vi "Data_SetEventRef.vi"(8 "error in (no error)":errorcluster, 10 "SendEventRef":T1) -> (0 "error out":errorcluster, 1 "ExtraLargeFile":bool, 2 "stream":bool, 3 "data":variant)   [LabVIEW 2017, in "FileManager.lvlib"]
uses:
  <vilib>/addons/InsightCM/Devices/Shared/Common/FileManager/FileManager.lvlib
  <vilib>/addons/InsightCM/Devices/Shared/Common/FileManager/controls/SendEventRefRoutedMessage.ctl
  <vilib>/addons/InsightCM/Devices/Shared/Common/DataEvent/controls/EventReference.ctl
  <vilib>/addons/InsightCM/Devices/Shared/Common/DataEvent/controls/Event.ctl
  <vilib>/addons/InsightCM/MessageBus/Base/controls/DataEvent.ctl
  <vilib>/addons/InsightCM/MessageBus/Base/controls/KeyValuePair.ctl
  <vilib>/addons/InsightCM/Devices/Shared/Common/DataEvent/controls/DataSet.ctl
  <vilib>/addons/InsightCM/MessageBus/Base/controls/DataSetMetadata.ctl
  <vilib>/addons/InsightCM/MessageBus/Base/controls/TrendPoint.ctl
  <vilib>/addons/InsightCM/MessageBus/Base/controls/TrendAlarmUpdate.ctl
  <vilib>/addons/InsightCM/MessageBus/Base/controls/TrendAlarmTransition.ctl
  <vilib>/addons/InsightCM/Devices/Shared/Common/FileManager/controls/DataPropertyNames.ctl
  <vilib>/addons/InsightCM/Devices/Shared/Common/FileManager/controls/DataType.ctl
  <vilib>/addons/InsightCM/Devices/Shared/Common/DataEvent/DataEvent.lvlib
panel:
  out "trend points only":bool
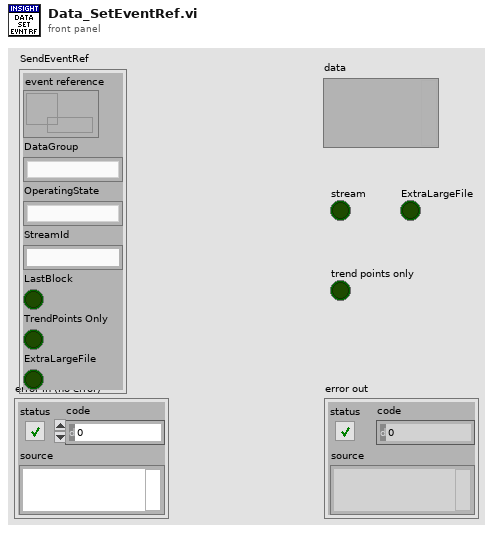
[diagram p1: front panel]
types:
  T1 = typedef "FileManager.lvlib/SendEventRefRoutedMessage.ctl" = cluster{"event reference":T2, "DataGroup":string, "OperatingState":string, "StreamId":string, "LastBlock":bool, "TrendPoints Only":bool, "ExtraLargeFile":bool}
  T2 = typedef "DataEvent.lvlib/EventReference.ctl" = refnum<data-value>
  T3 = typedef "DataPropertyNames.ctl" = enum16{"Type", "EventRef", "FilePath", "DataGroup", "AcquisitionTimestamp", "StreamId", "StreamBlock", "TrendPointsOnly", "ExtraLargeFile"}
  T4 = typedef "FileManager.lvlib/DataType.ctl" = enum16{"Default", "File", "InMemory", "EventRef", "EventRefFile"}
  T5 = typedef "DataEvent.lvlib/Event.ctl" = cluster{"DataEvent":T6, "DataSets":T8[], "TrendPoints":T10[], "Alarms":T11[]}
  T6 = typedef "DataEvent.ctl" = cluster{"Id":string, "AssetNodeId":string, "Timestamp":i64, "Props":T7[]}
  T7 = typedef "KeyValuePair.ctl" = cluster{"Key":string, "Value":string}
  T8 = typedef "DataEvent.lvlib/DataSet.ctl" = cluster{"DataSetMetadata":T9, "Values":sgl[], "Values DVR":refnum<data-value>}
  T9 = typedef "DataSetMetadata.ctl" = cluster{"Id":string, "DataEventId":string, "AssetNodeId":string, "Type":string, "T0":i64, "Props":T7[]}
  T10 = typedef "TrendPoint.ctl" = cluster{"TrendPointId":string, "DataEventId":string, "Timestamp":i64, "Value":dbl, "Props":T7[]}
  T11 = typedef "TrendAlarmUpdate.ctl" = cluster{"RuleId":string, "Transition":T12}
  T12 = typedef "TrendAlarmTransition.ctl" = cluster{"At":i64, "Severity":i32, "Value":dbl, "Properties":T7[]}
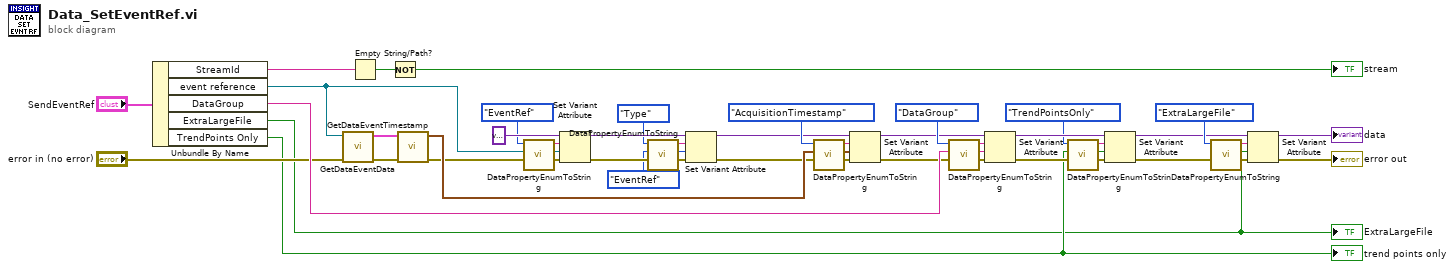
[diagram p0: block diagram]
diagram:
  n1 = Unbundle By Name("SendEventRef") -> ("StreamId"=w27:string, "event reference"=w21:T2, "DataGroup"=w33:string, "ExtraLargeFile"=w1:bool, "TrendPoints Only"=w2:bool)
  "trend points only" <- w2
  "ExtraLargeFile" <- w1
  n2 = call <vilib>:"GetDataEventData.vi"("error in (no error)"="error in (no error)", "Data Value Reference in"=w21) -> ("error out"=w22:errorcluster, "Data"=w20:T5)  [unwired: 8 in]
  n3 = Empty String/Path?(string/path=w27) -> (empty?=w26:bool)
  n4 = Not(x=w26) -> (.not. x?=→"stream":bool)
  n5 = call <vilib>:"GetDataEventTimestamp.vi"("error in (no error)"=w22, "data event"=w20) -> ("error out"=w24:errorcluster, "acquisition timestamp"=w30:timestamp)  [unwired: 8 in]
  n6 = call <vilib>:"DataPropertyEnumToString.vi"("property"=DataPropertyNames."EventRef" ("Names")) -> ("string"=w36:string)  [unwired: 10 in]
  n7 = Set Variant Attribute(Variant=variant ("DataInProgress"), name=w36, value=w21, error in=w24) -> (Variant out=w16:variant, error out=w19:errorcluster)  [unwired: 1 out]
  n8 = call <vilib>:"DataPropertyEnumToString.vi"("property"=DataPropertyNames."Type") -> ("string"=w15:string)  [unwired: 10 in]
  n9 = Set Variant Attribute(Variant=w16, name=w15, value=DataType."EventRef" ("DataType"), error in=w19) -> (Variant out=w17:variant, error out=w18:errorcluster)  [unwired: 1 out]
  n10 = call <vilib>:"DataPropertyEnumToString.vi"("property"=DataPropertyNames."AcquisitionTimestamp" ("Names")) -> ("string"=w31:string)  [unwired: 10 in]
  n11 = Set Variant Attribute(Variant=w17, name=w31, value=w30, error in=w18) -> (Variant out=w29:variant, error out=w28:errorcluster)  [unwired: 1 out]
  n12 = call <vilib>:"DataPropertyEnumToString.vi"("property"=DataPropertyNames."DataGroup" ("Names")) -> ("string"=w35:string)  [unwired: 10 in]
  n13 = Set Variant Attribute(Variant=w29, name=w35, value=w33, error in=w28) -> (Variant out=w11:variant, error out=w12:errorcluster)  [unwired: 1 out]
  n14 = call <vilib>:"DataPropertyEnumToString.vi"("property"=DataPropertyNames."TrendPointsOnly") -> ("string"=w10:string)  [unwired: 10 in]
  n15 = Set Variant Attribute(Variant=w11, name=w10, value=w2, error in=w12) -> (Variant out=w3:variant, error out=w6:errorcluster)  [unwired: 1 out]
  n16 = call <vilib>:"DataPropertyEnumToString.vi"("property"=DataPropertyNames."ExtraLargeFile") -> ("string"=w7:string)  [unwired: 10 in]
  n17 = Set Variant Attribute(Variant=w3, name=w7, value=w1, error in=w6) -> (Variant out=→"data":variant, error out=→"error out":errorcluster)  [unwired: 1 out]
